vi "03 Charts.vi"() -> ()   [LabVIEW 2019]
uses:
  _Subs/OpenDiagram/Open_XControl.xctl
panel:
  in  "OpenDiag":refnum<vi>(xcontrol)
  in  "stop":bool
  out "Chart":dbl(graph)
  in  "Slide":dbl(slide)=5.204081632653061 scale=0.0..10.0
  # "03 Charts\nThis code takes the value of the Slide and adds it to the Chart\n\nInstructions:\n1. Hit the Run arrow and see the Chart change as you change the value of the Slide\n2. Hit the STOP button to stop\n3. Right click on every control and indicator to see what you can change."
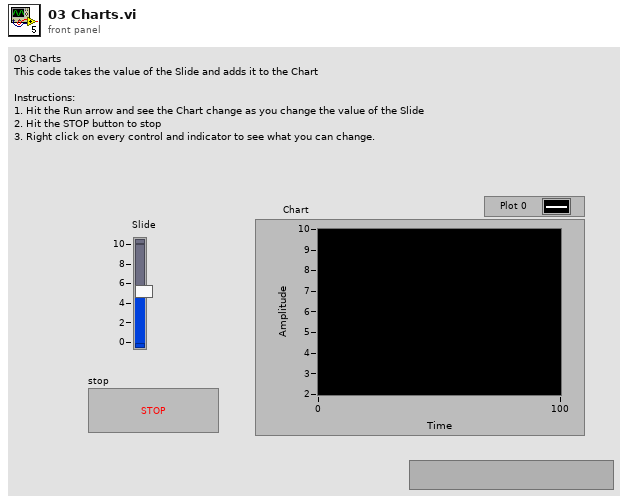
[diagram p1: front panel]
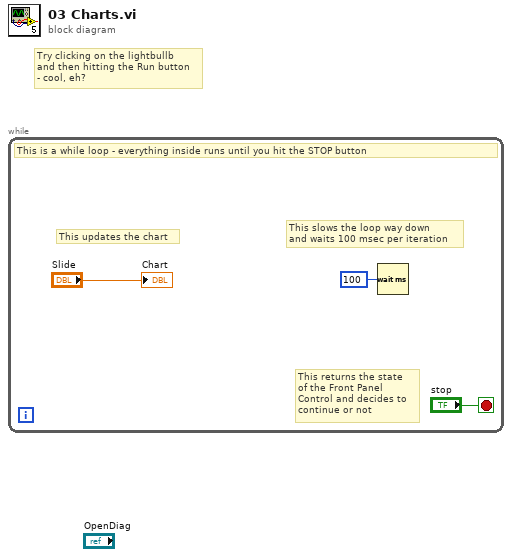
[diagram p0: block diagram]
diagram:
  # "Try clicking on the lightbullb\nand then hitting the Run button\n- cool, eh?"
  n1 = while {
    stop <- "stop" stop-if-true
    # "This returns the state\nof the Front Panel \nControl and decides to\ncontinue or not"
    # "This slows the loop way down \nand waits 100 msec per iteration"
    # "This updates the chart"
    # "This is a while loop - everything inside runs until you hit the STOP button"
    n2 = Wait (ms)(milliseconds to wait=u32 100) -> ()  [unwired: 1 out]
    "Chart" <- "Slide"
  }
